vi "RP-START SCPI.vi"(11 "RP IP":string="192.168.0.2") -> (3 "SCPI launched ?":bool)   [LabVIEW 2021]
uses:
  Field R&D Services/LIBSSH2 for LabVIEW/Toolkit/Session/Support/Create from SSH.vi
  Field R&D Services/LIBSSH2 for LabVIEW/Toolkit/Session/Support/Password Authentication.vi
  Field R&D Services/LIBSSH2 for LabVIEW/Toolkit/Channel/Support/Create from Session.vi
  Field R&D Services/LIBSSH2 for LabVIEW/Toolkit/Channel/Support/Destroy to Session.vi
  Field R&D Services/LIBSSH2 for LabVIEW/Toolkit/Session/Support/Destroy to SSH.vi
  Field R&D Services/LIBSSH2 for LabVIEW/Toolkit/SSH/SSH.lvclass
  Field R&D Services/LIBSSH2 for LabVIEW/Toolkit/Session/Session.lvclass
  Field R&D Services/LIBSSH2 for LabVIEW/Toolkit/Channel/Channel.lvclass
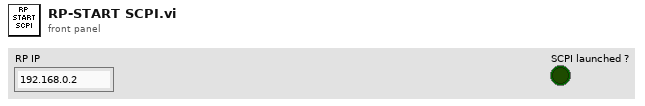
[diagram p1: front panel]
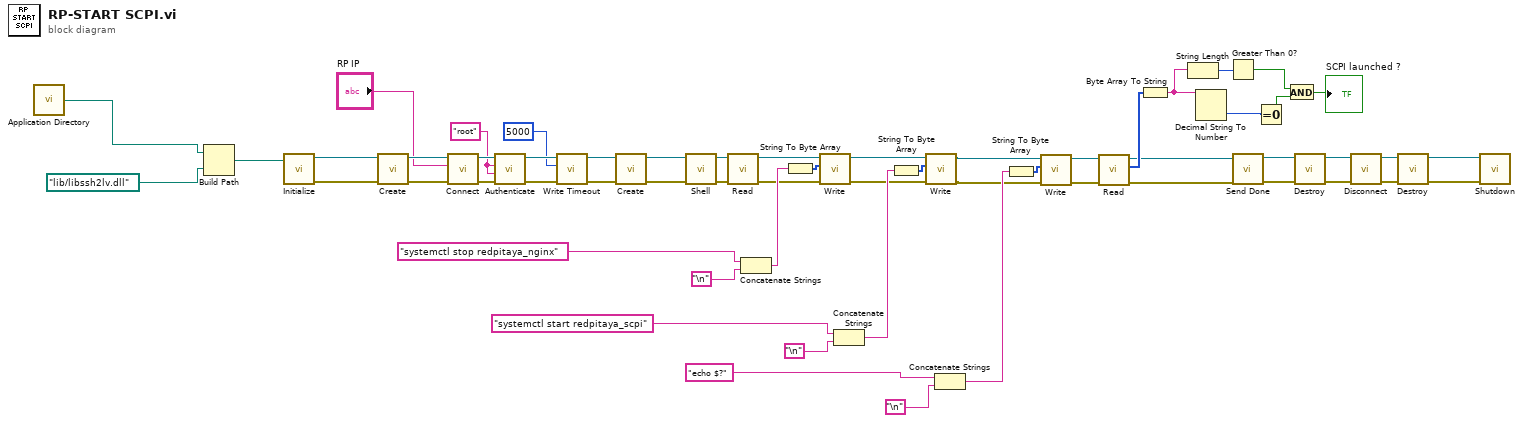
[diagram p0: block diagram]
diagram:
  w50 = "root" ("Username")
  n1 = call <vilib>:"Application Directory.vi"() -> ("Application Directory"=w2:path)
  n2 = Build Path(base path=w2, name or relative path=path "lib/libssh2lv.dll" ("libssh2lv Shared Library")) -> (appended path=w8:path)
  n3 = call "Initialize.vi"("libssh2lv Shared Library"=w8) -> ("Error Out"=w56:errorcluster, "SSH"=w57:refnum<class "SSH.lvclass">)  [unwired: 9 in]
  n4 = call-poly "Create.vi"("Error In"=w56, "SSH"=w57) -> ("Error Out"=w54:errorcluster, "Sesssion"=w55:refnum<class "Session.lvclass">)  [unwired: 8 in]
  n5 = call "Connect.vi"("Error In"=w54, "Address"="RP IP", "Session In"=w55) -> ("Error Out"=w51:errorcluster, "Sesssion Out"=w52:refnum<class "Session.lvclass">)  [unwired: 7 in]
  n6 = call-poly "Authenticate.vi"("Error In"=w51, "Password"=w50, "Username"=w50, "Session In"=w52) -> ("Error Out"=w41:errorcluster, "Sesssion Out"=w42:refnum<class "Session.lvclass">)  [unwired: 6 in]
  n7 = call "Write Timeout.vi"("Error In"=w41, "Timeout"=5000, "Session In"=w42) -> ("Error Out"=w40:errorcluster, "Sesssion Out"=w39:refnum<class "Session.lvclass">)  [unwired: 7 in]
  n8 = call-poly "Create.vi"("Error In"=w40, "Session"=w39) -> ("Error Out"=w48:errorcluster, "Channel"=w49:refnum<class "Channel.lvclass">)  [unwired: 8 in]
  n9 = call "Shell.vi"("Error In"=w48, "Channel In"=w49) -> ("Error Out"=w43:errorcluster, "Channel Out"=w44:refnum<class "Channel.lvclass">)  [unwired: 8 in]
  n10 = call "Read.vi"("Error In"=w43, "Channel In"=w44) -> ("Error Out"=w23:errorcluster, "Channel Out"=w24:refnum<class "Channel.lvclass">)  [unwired: 7 in, 1 out]
  n11 = Concatenate Strings("systemctl stop redpitaya_nginx", "\n") -> (w29:string)
  n12 = String To Byte Array(string=w29) -> (unsigned byte array=w45:u8[])
  n13 = call "Write.vi"("Error In"=w23, "Data"=w45, "Channel In"=w24) -> ("Error Out"=w21:errorcluster, "Channel Out"=w22:refnum<class "Channel.lvclass">)  [unwired: 6 in, 1 out]
  n14 = Concatenate Strings("systemctl start redpitaya_scpi", "\n") -> (w25:string)
  n15 = String To Byte Array(string=w25) -> (unsigned byte array=w28:u8[])
  n16 = call "Write.vi"("Error In"=w21, "Data"=w28, "Channel In"=w22) -> ("Error Out"=w17:errorcluster, "Channel Out"=w18:refnum<class "Channel.lvclass">)  [unwired: 6 in, 1 out]
  n17 = Concatenate Strings("echo $?", "\n") -> (w19:string)
  n18 = String To Byte Array(string=w19) -> (unsigned byte array=w20:u8[])
  n19 = call "Write.vi"("Error In"=w17, "Data"=w20, "Channel In"=w18) -> ("Error Out"=w14:errorcluster, "Channel Out"=w13:refnum<class "Channel.lvclass">)  [unwired: 6 in, 1 out]
  n20 = call "Read.vi"("Error In"=w14, "Channel In"=w13) -> ("Error Out"=w9:errorcluster, "Data"=w12:u8[], "Channel Out"=w10:refnum<class "Channel.lvclass">)  [unwired: 7 in]
  n21 = Byte Array To String(unsigned byte array=w12) -> (string=w7:string)
  n22 = String Length(string=w7) -> (length=w6:i32)
  n23 = Decimal String To Number(string=w7) -> (number=w11:i32)  [unwired: 2 in, 1 out]
  n24 = Greater Than 0?(x=w6) -> (x > 0?=w3:bool)
  n25 = call "Send Done.vi"("Error In"=w9, "Channel In"=w10) -> ("Error Out"=w32:errorcluster, "Channel Out"=w33:refnum<class "Channel.lvclass">)  [unwired: 8 in]
  n26 = Equal To 0?(x=w11) -> (x = 0?=w4:bool)
  n27 = And(x=w3, y=w4) -> (x .and. y?=→"SCPI launched ?":bool)
  n28 = call-poly "Destroy.vi"("Error In"=w32, "Channel"=w33) -> ("Error Out"=w35:errorcluster, "Session"=w34:refnum<class "Session.lvclass">)  [unwired: 8 in]
  n29 = call "Disconnect.vi"("Error In"=w35, "Session In"=w34) -> ("Error Out"=w36:errorcluster, "Sesssion Out"=w37:refnum<class "Session.lvclass">)  [unwired: 8 in]
  n30 = call-poly "Destroy.vi"("Error In"=w36, "Session"=w37) -> ("Error Out"=w46:errorcluster, "SSH"=w47:refnum<class "SSH.lvclass">)  [unwired: 8 in]
  n31 = call "Shutdown.vi"("Error In"=w46, "SSH"=w47) -> ()  [unwired: 9 in, 1 out]
